vi "Init.vi"(8 "error in (no error)":errorcluster, 10 "Instrument String":variant, 11 "NI Digitizer in":refnum<class "NI Digitizer.lvclass">) -> (0 "error out":errorcluster, 2 "Found?":bool, 3 "NI Digitizer out":refnum<class "NI Digitizer.lvclass">)   [LabVIEW 2025, in "Digitizer.lvlib" / "NI Digitizer.lvclass"]
uses:
  NI Digitizer.lvclass
  NI Digitizer.lvclass/NI Digitizer.ctl
  Digitizer Channel/Digitizer Channel.lvclass
  Digitizer Channel configuration/Digitizer Channel configuration.lvclass
  <vilib>/DAQmx/create/channels.llb/DAQmx Create Channel (AI-Voltage-Basic).vi
  Users/Public/Documents/Sandia National Labs/TSS Plugin/Abstract Engine.lvlibp/Plugin/Abstract/Abstract Instrument/Channel.ctl
  Users/Public/Documents/Sandia National Labs/TSS Plugin/Abstract Engine.lvlibp/Plugin/Abstract/Abstract Instrument/Abstract Instrument.lvclass
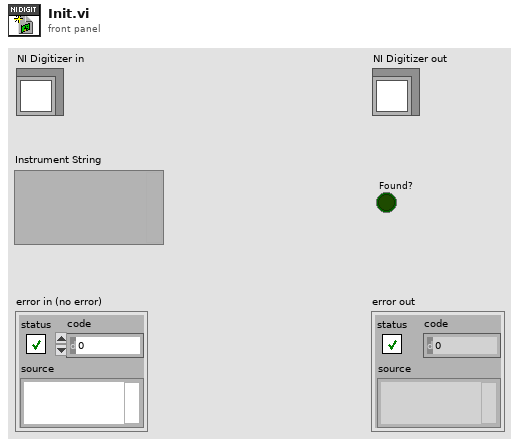
[diagram p1: front panel]
types:
  T1 = enum16{"---", "V", "A", "Ohm", "Hz", "uF", "degC", "deg"}
  T2 = typedef "Abstract Engine.lvlibp/Abstract Instrument.lvclass/Channel.ctl" = cluster{"Alias":string, "DataType":enum16{"Anaolg Input", "Waveform"}, "Unit":enum16{"---", "V", "A", "Ohm", "Hz", "uF", "degC", "deg"}, "Upper limit":dbl, "Lower limit":dbl, "Measurement":variant}
  T3 = typedef "Digitizer.lvlib/Digitizer Channel configuration.lvclass/Digitizer Channel Setting.ctl" = cluster{"Max":dbl, "Min":dbl, "Data Reduction":string, "Averging Points":u32, "Decimate Interval":u32, "Aperture Options":cluster{"Tolerance":u32, "Burst":u32, "Min SampleRate":u32, "Min SampleIndex":u32}}
  T4 = typedef "Abstract Engine.lvlibp/Channel configuration.lvclass/Default Channel.ctl" = cluster{"Address":string, "SW Alias":string, "Enabled":bool, "Type":string, "Description":string}
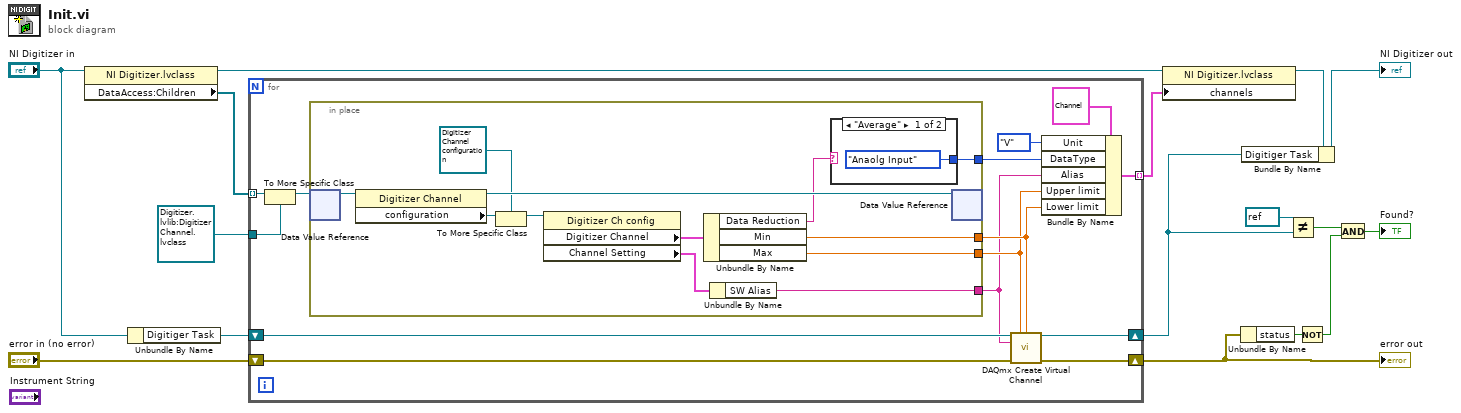
[diagram p0: block diagram]
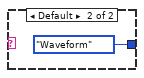
[diagram p2: hidden frame]
diagram:
  n1 = property class="NI Digitizer.lvclass"(reference="NI Digitizer in") -> (reference out=w12:refnum<class "NI Digitizer.lvclass">, "DataAccess:Children"=w4:refnum<data-value>[])  [unwired: 1 in, 1 out]
  n2 = Unbundle By Name("NI Digitizer in") -> ("Digitiger Task"=w5:refnum<k21>)
  n3 = for {
    shift-right: [w30] -> w10
    shift-left: "error in (no error)" -> [w22]
    shift-right: [w29] -> w13
    shift-left: w5 -> [w28]
    tunnel: w4 -> [w27] mode=indexing
    tunnel: [w25] -> w1 mode=indexing
    tunnel: refnum<data-value> refnum ("data value reference") -> [w23]
    n4 = To More Specific Class(target class=w23, reference=w27) -> (specific class reference=w26:refnum<data-value>)  [unwired: 1 in, 1 out]
    n5 = in-place {
      in-place-border: [w34] -> w20
      in-place-border: [w33] -> w19
      in-place-border: [w40] -> w18
      in-place-border: [w31] -> w17
      # "Initialize the front panel controls when loaded"
      n6 = in-place-dvr #1(w26) -> (w41:refnum<class "Digitizer Channel.lvclass">)  [unwired: 1 out]
      n7 = property class="Digitizer Channel"(reference=w41) -> (reference out=w42:refnum<class "Digitizer Channel.lvclass">, "configuration"=w39:refnum<class "CEF_serializable configuration.lvclass">)  [unwired: 1 in, 1 out]
      n8 = To More Specific Class(target class=refnum<class "Digitizer Channel configuration.lvclass"> refnum ("Digitizer.lvlib:Digitizer Channel configuration.lvclass"), reference=w39) -> (specific class reference=w38:refnum<class "Digitizer Channel configuration.lvclass">)  [unwired: 1 in, 1 out]
      n9 = property class="Digitizer Ch config"(reference=w38) -> ("Digitizer Channel"=w36:T3, "Channel Setting"=w35:T4)  [unwired: 1 in, 2 out]
      n10 = Unbundle By Name(w36) -> ("Data Reduction"=w32:string, "Min"=w34:dbl, "Max"=w33:dbl)
      n11 = Unbundle By Name(w35) -> ("SW Alias"=w40:string)
      n12 = case shown="\"Average\"" w32 {
        tunnel: [enum16{"Anaolg Input", "Waveform"}."Anaolg Input" ("DataType") enum16{"Anaolg Input", "Waveform"}."Waveform" ("DataType")] -> w31
        frame "Average" {
        }
        frame Default {
        }
      }
      n13 = in-place-dvr #1(w42) -> ()  [unwired: 2 out]
    }
    n14 = call-poly <vilib>:"DAQmx Create Virtual Channel.vi"("task in"=w28, "maximum value"=w19, "minimum value"=w20, "physical channels"=w18, "error in"=w22) -> ("task out"=w29:refnum<k21>, "error out"=w30:errorcluster)  [unwired: 9 in]
    n15 = Bundle By Name(cluster=T2 {"Alias"="ch0", "DataType"=enum."Anaolg Input", "Unit"=enum."V", "Upper limit"=10.0, "Lower limit"=-10.0, "Measurement"=variant} ("Channel"), "Unit"=T1."V", "DataType"=w17, "Alias"=w18, "Upper limit"=w19, "Lower limit"=w20) -> (w25:T2)
  }
  "error out" <- w10
  n16 = property class="NI Digitizer.lvclass"(reference=w12, "channels"=w1) -> (reference out=w2:refnum<class "NI Digitizer.lvclass">)  [unwired: 1 in, 1 out]
  n17 = Unbundle By Name(w10) -> ("status"=w11:bool)
  n18 = Bundle By Name(cluster=w2, "Digitiger Task"=w13) -> (→"NI Digitizer out":refnum<class "NI Digitizer.lvclass">)
  n19 = Not Equal?(x=refnum<k21> refnum, y=w13) -> (x != y?=w8:bool)
  n20 = Not(x=w11) -> (.not. x?=w9:bool)
  n21 = And(x=w8, y=w9) -> (x .and. y?=→"Found?":bool)
